vi "HVDD Lookup Table.vi"(11 "Lookup Table":string[][](array[string])) -> (3 "HVDD Voltage":string[][](array[string]))   [LabVIEW 2010]
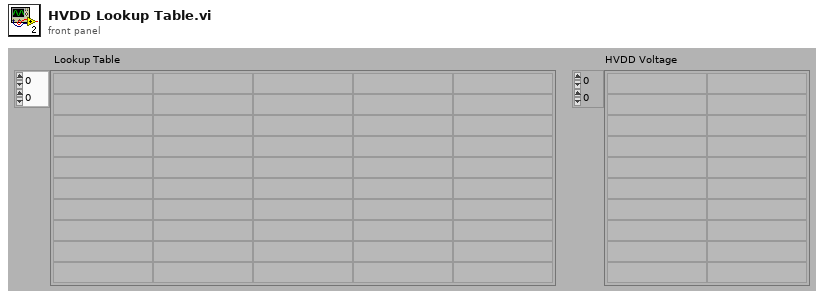
[diagram p1: front panel]
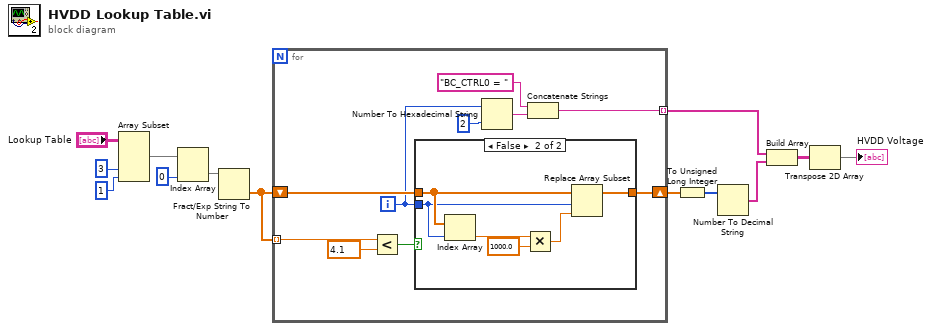
[diagram p0: block diagram]
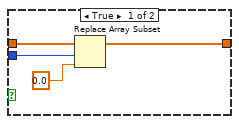
[diagram p2: hidden frame]
diagram:
  n1 = Array Subset(array="Lookup Table", index (col)=3 ("index"), length (col)=1 ("length")) -> (w10:string[][])  [unwired: 2 in]
  n2 = Index Array(array=w10, index (col)=0 ("index (row)")) -> (element=w8:string[])  [unwired: 1 in]
  n3 = Fract/Exp String To Number(string=w8) -> (number=w7:dbl[])  [unwired: 3 in, 1 out]
  n4 = for {
    tunnel: w7 -> [w23] mode=indexing
    shift-right: [w20] -> w6
    shift-left: w7 -> [w21]
    tunnel: [w15] -> w1 mode=indexing
    i -> [w18]
    n5 = Less?(x=w23, y=4.1) -> (x < y?=w22:bool)
    n6 = case shown="False" w22 {
      tunnel: w21 -> [w27 w32]
      tunnel: w18 -> [w26 w31]
      tunnel: [w25 w33] -> w20
      frame True {
        n7 = Replace Array Subset(array=w27, new element=0.0 ("new element/subarray"), index=w26) -> (w25:dbl[])
      }
      frame False {
        n8 = Index Array(array=w32, index=w31) -> (element=w29:dbl)
        n9 = Multiply(x=w29, y=1000.0) -> (x*y=w28:dbl)
        n10 = Replace Array Subset(array=w32, new element=w28, index=w31) -> (w33:dbl[])
      }
    }
    n11 = Number To Hexadecimal String(1:i16 2 ("width (-)"), 2:w18) -> (0:w16:string)
    n12 = Concatenate Strings("BC_CTRL0 = " ("hex integer string"), w16) -> (w15:string)
  }
  n13 = To Unsigned Long Integer(number=w6) -> (unsigned 32bit integer=w5:u32[])
  n14 = Number To Decimal String(number=w5) -> (decimal integer string=w4:string[])  [unwired: 1 in]
  n15 = Build Array(w1, w4) -> (w3:string[][])
  n16 = Transpose 2D Array(2D array=w3) -> (transposed array=→"HVDD Voltage":string[][])
